vi "3DLDA_Pre_Analysis_Plugin.vi"() -> ()   [LabVIEW 2020]
uses:
  <vilib>/Analysis/baseanly.llb/A x Vector.vi
  Globals/LDA_global.vi
  Globals/Meas_global.vi
  Globals/Constants_global.vi
  <vilib>/Analysis/NI_AALBase.lvlib
panel:
  in  "Plot Data":bool
  out "XY Graph":cluster{"Time (s)":dbl[], dbl[]}[](graph)
  out "error":i32
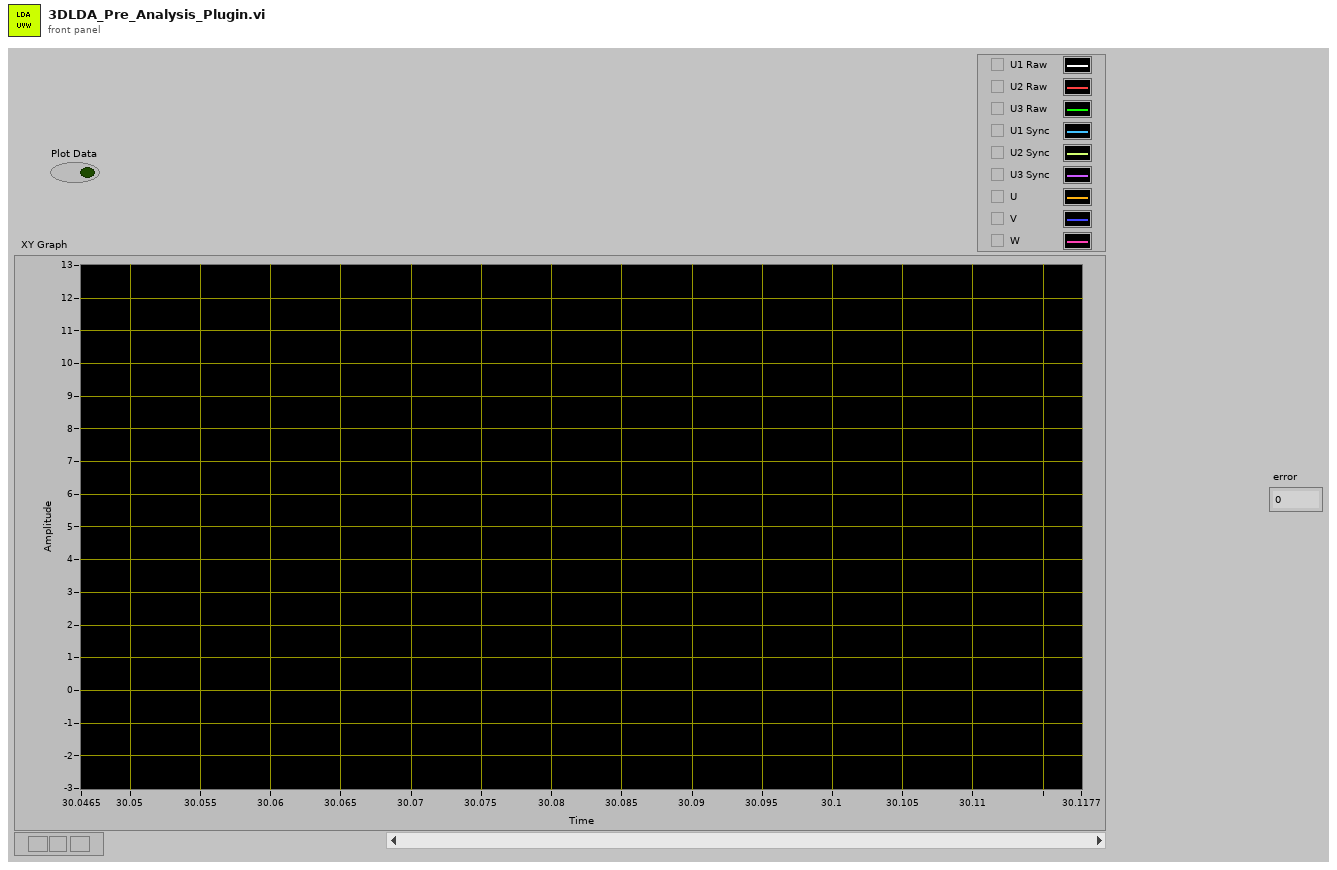
[diagram p1: front panel]
types:
  T1 = typedef "Analysis_info_cluster.ctl" = cluster{"Colour":u32, "Inst type":T2, "Inst name":string, "Symbol":string, "Code name":string, "Extra Info":string, "Inst Array":T3, "Extra Titles":string[], "Extra Values":string[], "U":dbl, "u^2":dbl, "u^3":dbl, "u^4":dbl, "Skew_u":dbl, "Kurt_u":dbl, "Sd Error in Mean":dbl, "% u'/U":dbl, "X":dbl, "Y":dbl, "Z":dbl, "Timescale integral Estimate":dbl, "Sd Error in Variance":dbl, "Calib File":path, "Calib Constants":dbl[], "Output Position":bool, "Stats":enum16{"None", "Basic", "Full"}, "Av Sampling Rate":dbl, "Av No of Samples":dbl, "Total Meas Time (s)":dbl, "ADAM Ch Name":string, "Max value":dbl, "Min value":dbl, "Req Sample Rate Hz":dbl, "Sync Delay Time (s)":dbl, "Ch No":i16, "Device":string, "Use Latest Calib":bool, "Port":string, "Metadata Ch Names":string[], "Metadata Ch Values":string[], "Label":string}
  T2 = typedef "Inst_type.ctl" = enum16{"Propeller anemometer", "Raw voltage", "Pressure Transducer", "Pitot-static tube", "Hot wire", "Cross wire 1", "Cross wire 2", "Generic Linear", "Generic Polynomial", "Generic BackPoly", "Fast FID", "Thermocouple", "Cold wire", "Pulsed Wire", "LDA Vel", "LDA Tran time", "LDA Arr time", "Microphone"}
  T3 = typedef "Instrument_Array.ctl" = enum16{"PWA", "LDA", "Analogue"}
  T4 = typedef "Time_Trace_Cluster.ctl" = cluster{"Weighting":dbl[], "Time (s)":dbl[], "Voltage":dbl[], "Eng Values":dbl[]}
  T5 = typedef "NI_Matrix.lvlib/RealMatrix.ctl" = dbl[][]
  T6 = enum16{"X Axis Fixed", "Y Axis Fixed", "Z Axis Fixed"}
  T7 = typedef "Cross_Moments_Shift_Cluster.ctl" = cluster{"Stats":dbl[], "Resampled No of Samples":i32, "Resampled delta T":dbl, "Cross Correlation":dbl[]}
  T8 = typedef "Shift_Cluster.ctl" = cluster{"Stats":dbl[], "Spectra_Auto":dbl[], "Histogram":dbl[], "Hist Max":dbl, "Hist Min":dbl, "No of Samples":i32, "No in plume":i32, "Weight sum":dbl, "No Of Hist bins":i32, "TimeTrace Max":dbl, "Time Trace Min":dbl, "Trace St Deviation":dbl}
  T9 = typedef "Correlation_cluster1.ctl" = cluster{"U inst":string, "uw":dbl, "u^2w":dbl, "uw^2":dbl, "uw/u'w'":dbl, "W inst":string, "uw^3":dbl, "u^3w":dbl, "u^2w^2":dbl, "Index U":i32, "Index W":i32, "Error info":string[], "Paired Sampling Rate (Hz)":dbl, "u^2 Paired":dbl, "w^2 Paired":dbl, "Time Window (ms)":dbl}
  T10 = typedef "Post_Process.ctl" = enum16{"Take New Data", "Post Process Raw Data File"}
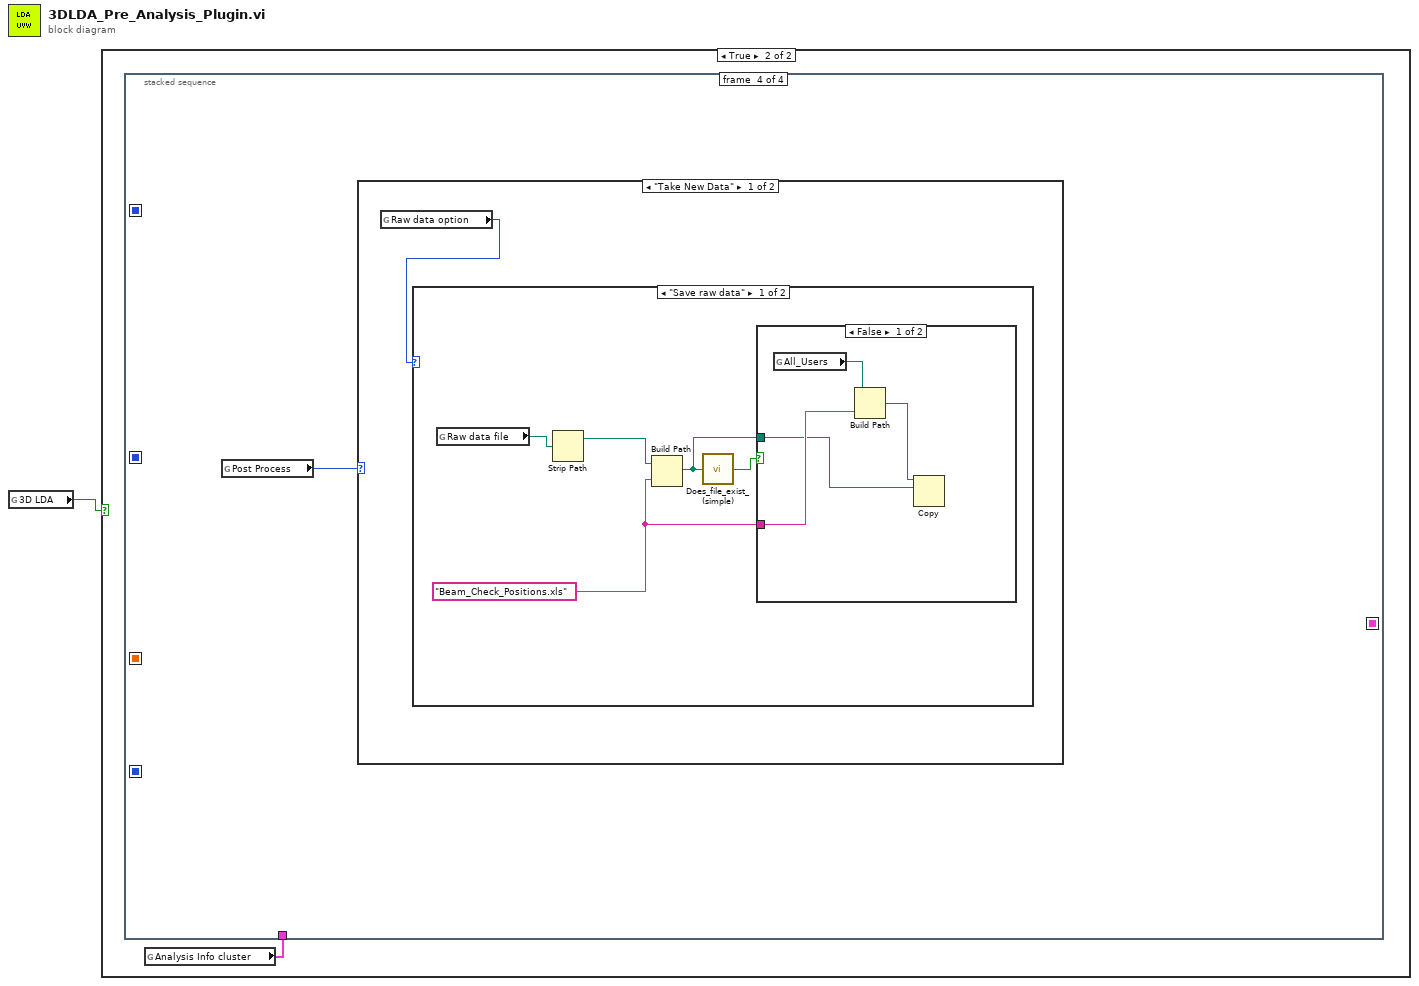
[diagram p0: block diagram]
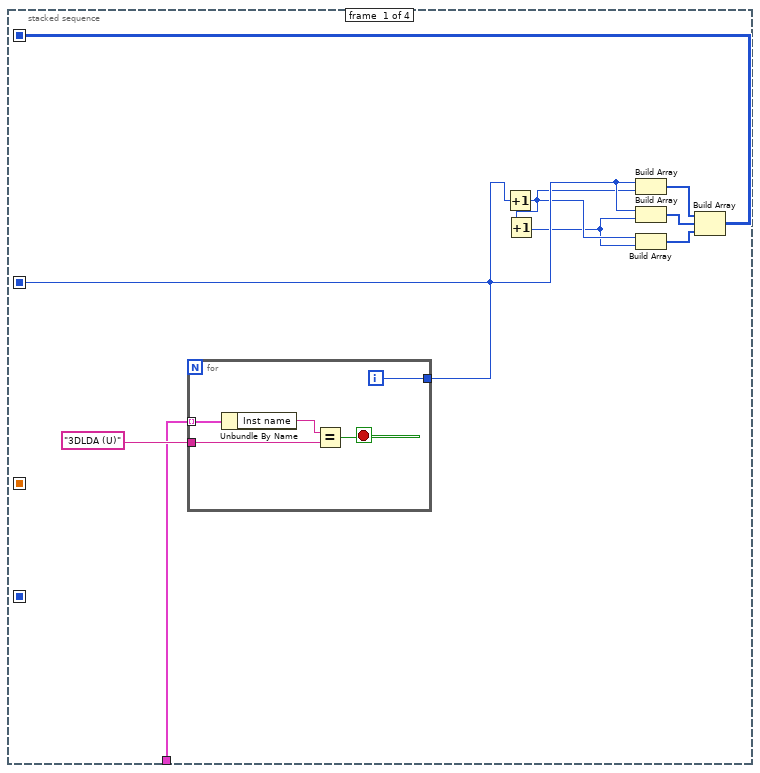
[diagram p3: hidden frame]
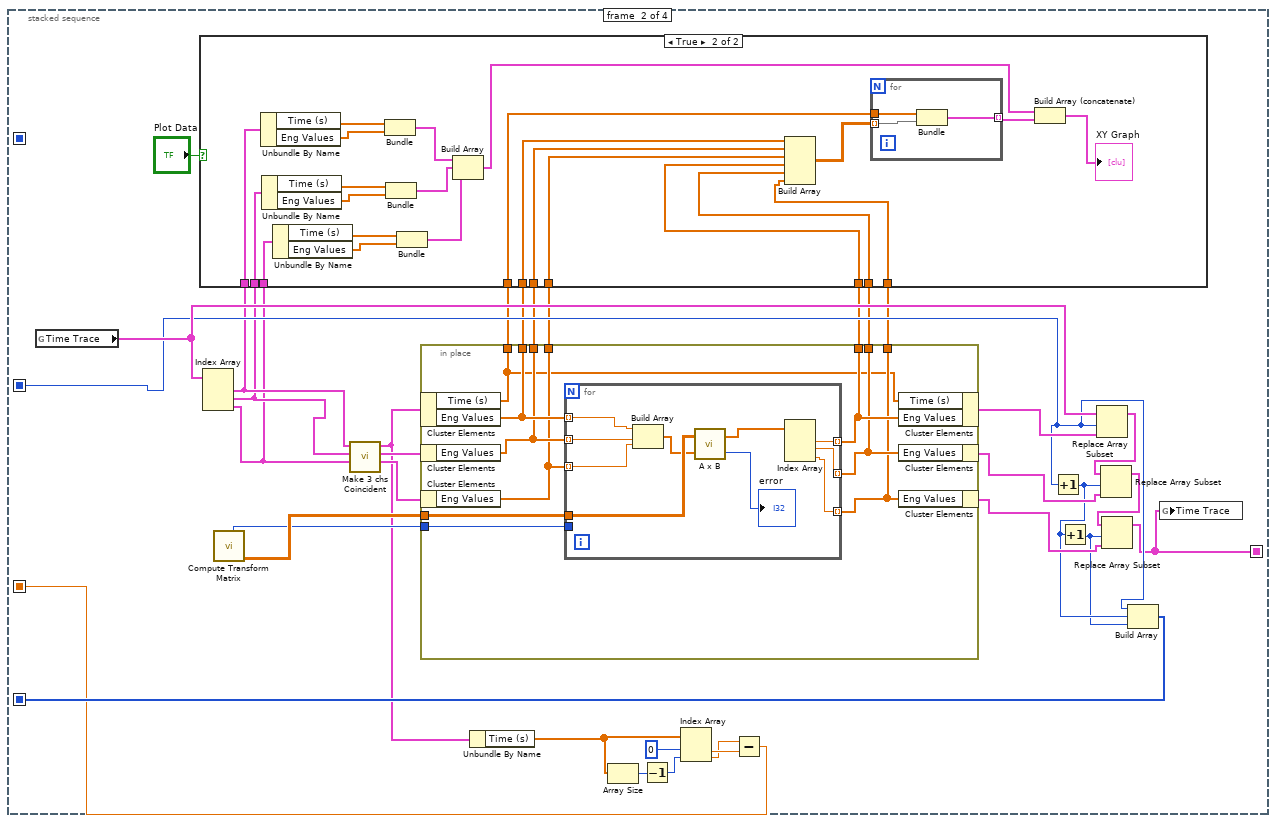
[diagram p4: hidden frame]
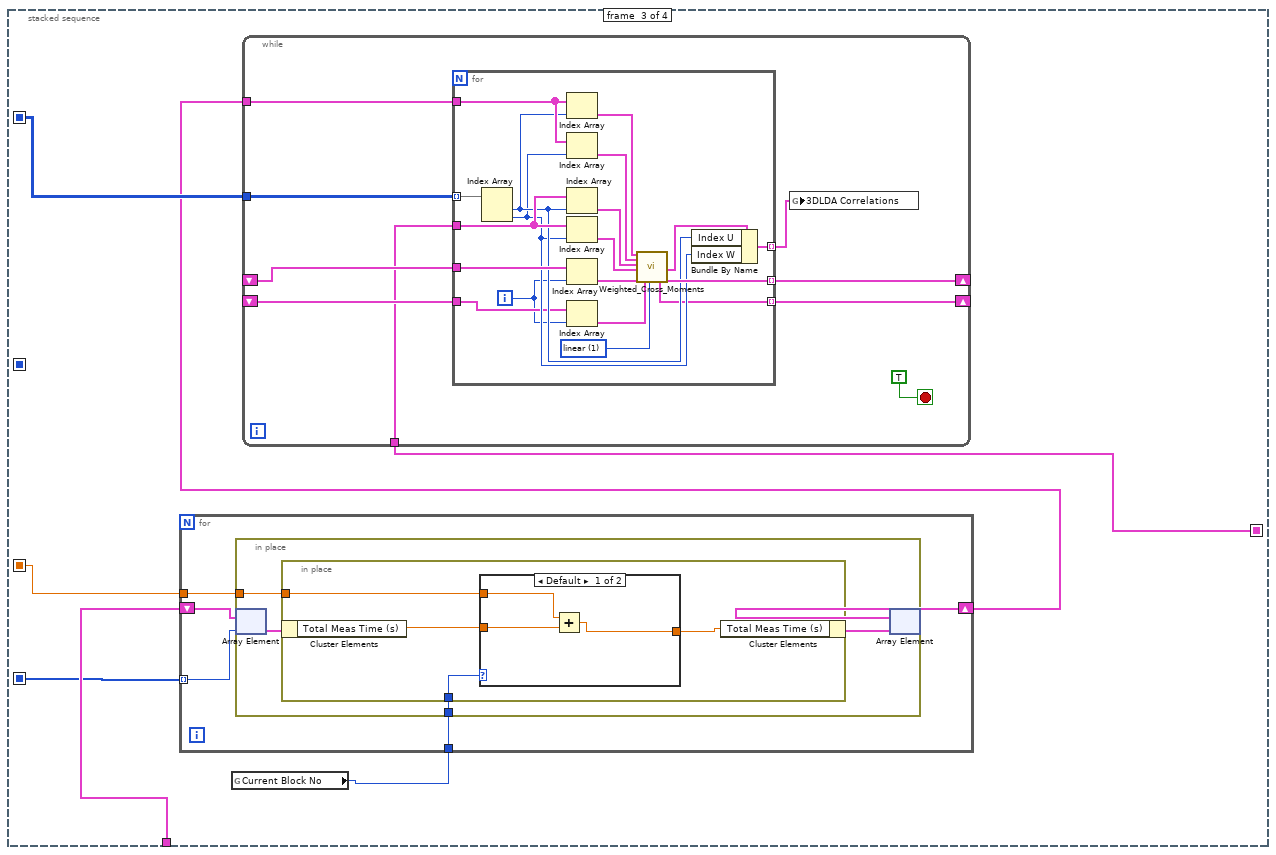
[diagram p6: hidden frame]
diagram:
  n1 = global read "LDA_global.vi" "3D LDA"() -> (w1:bool)
  n2 = case shown="True" w1 {
    frame False {
    }
    frame True {
      n3 = global read "Meas_global.vi" "Analysis Info cluster"() -> (w2:T1[])
      n4 = stacked-sequence {
        seq-local: [w11 _ _ _] -> [_ _ w102 _]
        seq-local: [w6 _ _ _] -> [_ w41 _ _]
        seq-local: [_ w29 _ _] -> [_ _ w97 _]
        seq-local: [_ w38 _ _] -> [_ _ w100 _]
        seq-local: [_ w18 _ _] -> [_ _ w96 _]
        tunnel: w2 -> [w3 _ w101 _]
        frame #0 {
          n5 = for {
            tunnel: w3 -> [w16] mode=indexing
            tunnel: "3DLDA (U)" ("format string") -> [w14]
            tunnel: [w12] -> w6
            i -> [w12]
            stop <- w13 stop-if-true
            n6 = Unbundle By Name(w16) -> ("Inst name"=w15:string)
            n7 = Equal?(x=w15, y=w14) -> (x = y?=w13:bool)
          }
          n8 = Increment(x=w6) -> (x+1=w5:i32)
          n9 = Increment(x=w5) -> (x+1=w4:i32)
          n10 = Build Array(w6, w5) -> (w8:i32[])
          n11 = Build Array(w6, w4) -> (w9:i32[])
          n12 = Build Array(w5, w4) -> (w10:i32[])
          n13 = Build Array(w8, w9, w10) -> (w11:i32[][])
        }
        frame #1 {
          n14 = global read "Meas_global.vi" "Time Trace"() -> (w48:T4[])
          n15 = Index Array(array=w48) -> (element #1=w21:T4, element #2=w20:T4, element #3=w19:T4)  [unwired: 3 in]
          n16 = call "Compute Transform Matrix.vi"() -> ("Inverse Matrix"=w43:T5, "Fixed Axis"=w42:T6)  [unwired: 6 in, 4 out]
          n17 = call "Make 3 chs Coincident.vi"("Time Cluster 3"=w19, "Time Cluster 2"=w20, "Time Cluster 1"=w21) -> ("Coincident Time Cluster 3"=w32:T4, "Coincident Time Cluster 2"=w47:T4, "Coincident Time Cluster 1"=w31:T4)  [unwired: 6 in]
          n18 = in-place {
            in-place-border: w43 -> [w85]
            in-place-border: w42 -> [w84]
            in-place-border: [w83] -> w28
            in-place-border: [w82] -> w27
            in-place-border: [w81] -> w26
            in-place-border: [w80] -> w25
            in-place-border: [w79] -> w24
            in-place-border: [w78] -> w23
            in-place-border: [w77] -> w22
            n19 = in-place-cluster #1(w31) -> ("Time (s)"=w77:dbl[], "Eng Values"=w83:dbl[])
            n20 = in-place-cluster #2(w47) -> ("Eng Values"=w82:dbl[])
            n21 = in-place-cluster #3(w32) -> ("Eng Values"=w81:dbl[])
            n22 = for {
              tunnel: w83 -> [w95] mode=indexing
              tunnel: w82 -> [w94] mode=indexing
              tunnel: w81 -> [w93] mode=indexing
              tunnel: w85 -> [w88]
              tunnel: [w92] -> w80 mode=indexing
              tunnel: [w91] -> w79 mode=indexing
              tunnel: [w90] -> w78 mode=indexing
              tunnel: w84 -> [_]
              n23 = Build Array(w95, w94, w93) -> (w87:dbl[])
              n24 = call-poly <vilib>:"A x B.vi"("Vector"=w87, "A"=w88) -> ("error"=→"error":i32, "A x Vector"=w86:dbl[])
              n25 = Index Array(array=w86) -> (element #1=w92:dbl, element #2=w91:dbl, element #3=w90:dbl)  [unwired: 3 in]
            }
            n26 = in-place-cluster #1("Time (s)"=w77, "Eng Values"=w80) -> (w46:T4)
            n27 = in-place-cluster #2("Eng Values"=w79) -> (w45:T4)
            n28 = in-place-cluster #3("Eng Values"=w78) -> (w44:T4)
          }
          n29 = case shown="True" "Plot Data" {
            tunnel: w28 -> [_ w73]
            tunnel: w27 -> [_ w72]
            tunnel: w26 -> [_ w71]
            tunnel: w25 -> [_ w70]
            tunnel: w24 -> [_ w69]
            tunnel: w23 -> [_ w68]
            tunnel: w22 -> [_ w67]
            tunnel: w21 -> [_ w65]
            tunnel: w20 -> [_ w58]
            tunnel: w19 -> [_ w57]
            frame False {
            }
            frame True {
              n30 = Unbundle By Name(w65) -> ("Time (s)"=w64:dbl[], "Eng Values"=w63:dbl[])
              n31 = Unbundle By Name(w58) -> ("Time (s)"=w61:dbl[], "Eng Values"=w62:dbl[])
              n32 = Unbundle By Name(w57) -> ("Time (s)"=w60:dbl[], "Eng Values"=w59:dbl[])
              n33 = Bundle("Time (s)"=w64, "Eng Values"=w63) -> (w56:cluster{"Time (s)":dbl[], "Eng Values":dbl[]})  [unwired: 1 in]
              n34 = Bundle("Time (s)"=w61, "Eng Values"=w62) -> (w55:cluster{"Time (s)":dbl[], "Eng Values":dbl[]})  [unwired: 1 in]
              n35 = Bundle("Time (s)"=w60, "Eng Values"=w59) -> (w54:cluster{"Time (s)":dbl[], "Eng Values":dbl[]})  [unwired: 1 in]
              n36 = Build Array(w56, w55, w54) -> (w53:cluster{"Time (s)":dbl[], "Eng Values":dbl[]}[])
              n37 = Build Array(w73, w72, w71, w70, w69, w68) -> (w66:dbl[][])
              n38 = for {
                tunnel: w67 -> [w76]
                tunnel: w66 -> [w75] mode=indexing
                tunnel: [w74] -> w52 mode=indexing
                n39 = Bundle("Time (s)"=w76, w75) -> (w74:cluster{"Time (s)":dbl[], dbl[]})  [unwired: 1 in]
              }
              n40 = Build Array (concatenate)(w53, w52) -> (→"XY Graph":cluster{"Time (s)":dbl[], "Eng Values":dbl[]}[])
            }
          }
          n41 = Unbundle By Name(w31) -> ("Time (s)"=w30:dbl[])
          n42 = Array Size(array=w30) -> (size(s)=w35:i32)
          n43 = Decrement(x=w35) -> (x-1=w34:i32)
          n44 = Index Array(array=w30, index #1=0 ("index"), index #2=w34) -> (element #1=w37:dbl, element #2=w36:dbl)
          n45 = Subtract(x=w36, y=w37) -> (x-y=w29:dbl)
          n46 = Increment(x=w41) -> (x+1=w40:i32)
          n47 = Increment(x=w40) -> (x+1=w39:i32)
          n48 = Replace Array Subset(array=w48, new element=w46, index=w41) -> (w49:T4[])
          n49 = Replace Array Subset(array=w49, new element=w45, index=w40) -> (w50:T4[])
          n50 = Replace Array Subset(array=w50, new element=w44, index=w39) -> (w18:T4[])
          n51 = Build Array(w41, w40, w39) -> (w38:i32[])
          n52 = global write "Meas_global.vi" "Time Trace"(w18) -> ()
        }
        frame #2 {
          n53 = global read "Meas_global.vi" "Current Block No"() -> (w98:i32)
          n54 = for {
            shift-right: [w105] -> w99
            shift-left: w101 -> [w107]
            tunnel: w100 -> [w106] mode=indexing
            tunnel: w98 -> [w104]
            tunnel: w97 -> [w103]
            n55 = in-place {
              in-place-border: w104 -> [w109]
              in-place-border: w103 -> [w108]
              n56 = in-place-array #4(w107, w106) -> (w111:T1)
              n57 = in-place {
                in-place-border: w109 -> [w115]
                in-place-border: w108 -> [w113]
                n58 = in-place-cluster #5(w111) -> ("Total Meas Time (s)"=w112:dbl)
                n59 = case shown="Default" w115 {
                  tunnel: [w116 w119] -> w114
                  tunnel: w113 -> [w118 w119]
                  tunnel: w112 -> [w117 _]
                  frame Default {
                    n60 = Add(x=w118, y=w117) -> (x+y=w116:dbl)
                  }
                  frame 1 {
                  }
                }
                n61 = in-place-cluster #5("Total Meas Time (s)"=w114) -> (w110:T1)
              }
              n62 = in-place-array #4(w110) -> (w105:T1[])  [unwired: 1 out]
            }
          }
          n63 = while {
            shift-right: [w128] -> _
            shift-left: _ -> [w126]
            shift-right: [w127] -> _
            shift-left: _ -> [w125]
            tunnel: w102 -> [w124]
            tunnel: w99 -> [w121]
            tunnel: w96 -> [w120]
            stop <- TRUE stop-if-true
            n64 = for {
              tunnel: w124 -> [w147] mode=indexing
              tunnel: w121 -> [w145]
              tunnel: [w143] -> w128 mode=indexing
              tunnel: w126 -> [w142]
              tunnel: [w139] -> w122 mode=indexing
              tunnel: w120 -> [w138]
              tunnel: [w131] -> w127 mode=indexing
              tunnel: w125 -> [w130]
              i -> [w129]
              w133 = 1 items=["nearest", "linear", "spline", "cubic Hermite", "Lagrange"] ("interp. method")
              n65 = Index Array(array=w147) -> (element #1=w137:i32, element #2=w136:i32)  [unwired: 2 in]
              n66 = Index Array(array=w145, index=w137) -> (element=w146:T1)
              n67 = Index Array(array=w145, index=w136) -> (element=w144:T1)
              n68 = Index Array(array=w138, index=w137) -> (element=w135:T4)
              n69 = Index Array(array=w138, index=w136) -> (element=w134:T4)
              n70 = Index Array(array=w142, index=w129) -> (element=w141:T7)
              n71 = Index Array(array=w130, index=w129) -> (element=w132:T8)
              n72 = call "Weighted_Cross_Moments.vi"("AI Cluster 1"=w146, "AI Cluster 2"=w144, "Time Cluster 1"=w135, "Time Cluster 2"=w134, "Shift Cluster In"=w141, "Shift Input"=w132, "interp. method"=w133) -> ("Shift Output"=w131:T8, "output cluster"=w140:T9, "Shift Cluster Out"=w143:T7)  [unwired: 10 in]
              n73 = Bundle By Name(cluster=w140, "Index U"=w137, "Index W"=w136) -> (w139:T9)
            }
            n74 = global write "LDA_global.vi" "3DLDA Correlations"(w122) -> ()
          }
        }
        frame #3 {
          n75 = global read "Meas_global.vi" "Post Process"() -> (w148:T10)
          n76 = case shown="\"Take New Data\"" w148 {
            frame "Take New Data" {
              n77 = global read "Meas_global.vi" "Raw data option"() -> (w149:enum16{"Save raw data", "Raw data not saved"})
              n78 = case shown="\"Save raw data\"" w149 {
                frame "Save raw data" {
                  w151 = "Beam_Check_Positions.xls" ("Substring")
                  n79 = global read "Meas_global.vi" "Raw data file"() -> (w154:path)
                  n80 = Strip Path(path=w154) -> (stripped path=w153:path)  [unwired: 1 out]
                  n81 = Build Path(base path=w153, name or relative path=w151) -> (appended path=w150:path)
                  n82 = call "Does_file_exist_(simple).vi"("Pathname"=w150) -> ("exists?"=w152:bool)
                  n83 = case shown="False" w152 {
                    tunnel: w151 -> [w157 _]
                    tunnel: w150 -> [w155 _]
                    frame False {
                      n84 = global read "Constants_global.vi" "All_Users"() -> (w158:path)
                      n85 = Build Path(base path=w158, name or relative path=w157) -> (appended path=w156:path)
                      n86 = Copy(10:w155, 11:w156) -> ()  [unwired: 3 in, 3 out]
                    }
                    frame True {
                    }
                  }
                }
                frame "Raw data not saved" {
                }
              }
            }
            frame "Post Process Raw Data File" {
            }
          }
        }
      }
    }
  }
